vi "Set LakeShore 340 Heater Range.vi"(8 "error in (no error)":errorcluster, 10 "Set Heater Range":T1, 11 "VISA resource name":refnum<visa-resource-name>) -> (0 "error out":errorcluster, 3 "VISA resource name out":refnum<visa-resource-name>)   [LabVIEW 2015]
uses:
  LakeShore340 Heater Ranges.ctl
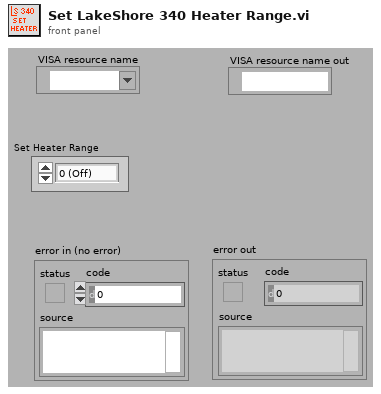
[diagram p1: front panel]
types:
  T1 = typedef "LakeShore340 Heater Ranges.ctl" = enum16{"0 (Off)", "1 (5 mW)", "2 (50 mW)", "3 (500 mW)", "4 (5 W)", "5 (50 W)"}
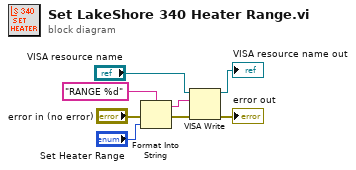
[diagram p0: block diagram]
diagram:
  n1 = Format Into String(format string="RANGE %d" ("write buffer"), error in="error in (no error)", "Set Heater Range") -> (resulting string=w6:string, error out=w7:errorcluster)  [unwired: 1 in]
  n2 = VISA Write(VISA resource name="VISA resource name", write buffer=w6, error in (no error)=w7) -> (VISA resource name out=→"VISA resource name out":refnum<visa-resource-name>, error out=→"error out":errorcluster)  [unwired: 1 out]
